vi "Ramp.vi"(1 "Max Deccel (Vs/ms)":dbl, 2 "Input":dbl, 3 "Max Accel (Vs/ms)":dbl) -> (0 "Output":dbl)   [LabVIEW 2014]
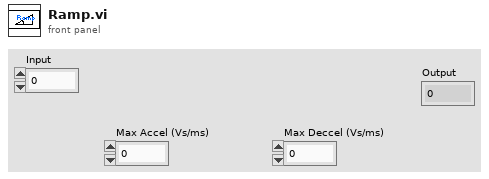
[diagram p1: front panel]
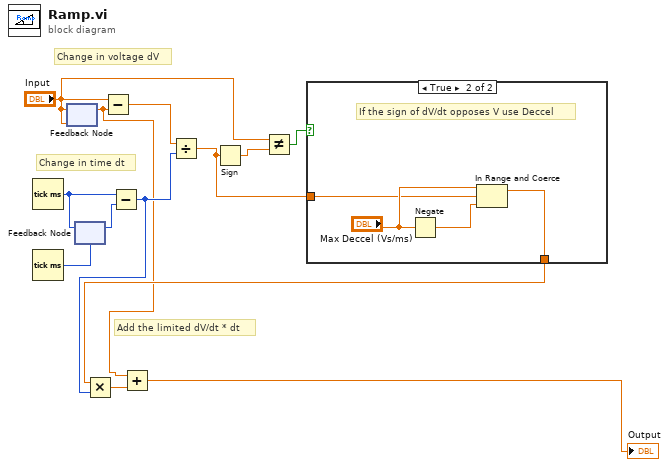
[diagram p0: block diagram]
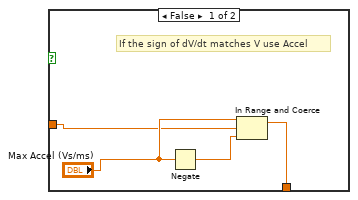
[diagram p2: hidden frame]
diagram:
  # "Add the limited dV/dt * dt"
  # "Change in time dt"
  # "Change in voltage dV"
  n1 = Tick Count (ms)() -> (millisecond timer value=w11:u32)
  n2 = Tick Count (ms)() -> (millisecond timer value=w13:u32)
  n3 = feedback-in #1("Input") -> ()
  n4 = feedback #1("Input") -> (w2:dbl)
  n5 = feedback-in #2(w11) -> ()
  n6 = feedback #2(w13) -> (w12:u32)
  n7 = Subtract(x="Input", y=w2) -> (x-y=w10:dbl)
  n8 = Subtract(x=w11, y=w12) -> (x-y=w3:u32)
  n9 = Divide(x=w10, y=w3) -> (x/y=w6:dbl)
  n10 = Sign(1:w6) -> (0:w9:dbl)
  n11 = Not Equal?(x="Input", y=w9) -> (x != y?=w7:bool)
  n12 = case shown="True" w7 {
    tunnel: w6 -> [w15 w19]
    tunnel: [w14 w18] -> w4
    frame False {
      # "If the sign of dV/dt matches V use Accel"
      n13 = Negate(x="Max Accel (Vs/ms)") -> (-x=w17:dbl)
      n14 = In Range and Coerce(upper limit="Max Accel (Vs/ms)", x=w15, lower limit=w17) -> (coerced(x)=w14:dbl)  [unwired: 1 out]
    }
    frame True {
      # "If the sign of dV/dt opposes V use Deccel"
      n15 = Negate(x="Max Deccel (Vs/ms)") -> (-x=w21:dbl)
      n16 = In Range and Coerce(upper limit="Max Deccel (Vs/ms)", x=w19, lower limit=w21) -> (coerced(x)=w18:dbl)  [unwired: 1 out]
    }
  }
  n17 = Multiply(x=w4, y=w3) -> (x*y=w5:dbl)
  n18 = Add(x=w2, y=w5) -> (x+y=→"Output":dbl)
